vi "QueryMirror.vi"(8 "error in (no error)":errorcluster, 10 "Mirror":enum16{"Entrance Mirror", "Exit Mirror"}(ring), 11 "HRS_Spectrometer in":refnum<class "HRS_Spectrometer.lvclass">) -> (0 "error out":errorcluster, 3 "HRS_Spectrometer out":refnum<class "HRS_Spectrometer.lvclass">)   [LabVIEW 2023, in "HRS_Spectrometer.lvlib" / "HRS_Spectrometer.lvclass"]
uses:
  HRS_Spectrometer.lvclass
  HRS_Spectrometer.lvclass/HRS_Spectrometer.ctl
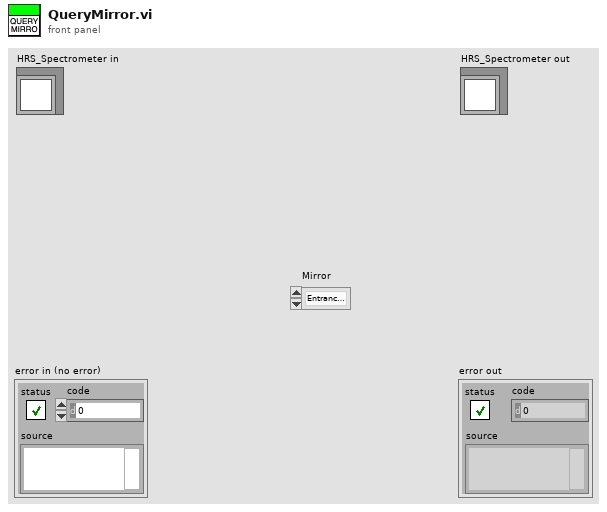
[diagram p1: front panel]
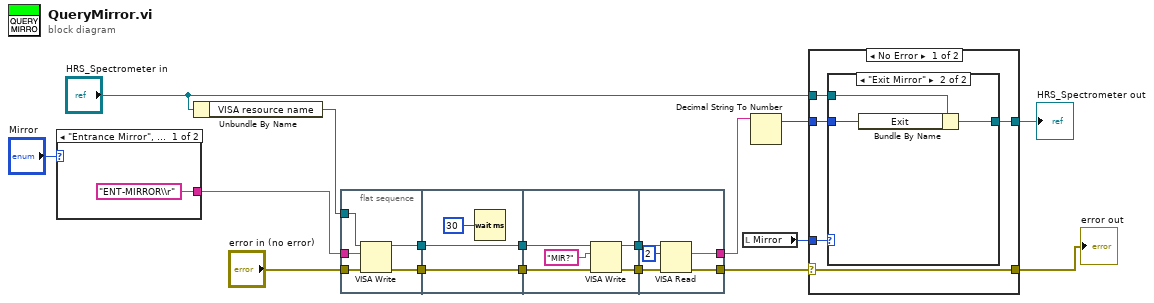
[diagram p0: block diagram]
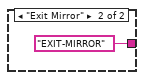
[diagram p2: hidden frame]
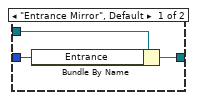
[diagram p3: hidden frame]
diagram:
  n1 = case shown="\"Entrance Mirror\", Default" "Mirror" {
    tunnel: ["ENT-MIRROR\\r" ("write buffer") "EXIT-MIRROR" ("write buffer")] -> w9
    frame "Entrance Mirror", Default {
    }
    frame "Exit Mirror" {
    }
  }
  n2 = Unbundle By Name("HRS_Spectrometer in") -> ("VISA resource name"=w11:refnum<visa-resource-name>)
  n3 = flat-sequence {
    tunnel: [w24] -> w17
    tunnel: [w23] -> w16
    tunnel: w11 -> [w22]
    tunnel: "error in (no error)" -> [w21]
    tunnel: w9 -> [w20]
    tunnel: w17 -> [w27]
    tunnel: w16 -> [w26]
    tunnel: [w27] -> w8
    tunnel: [w26] -> w6
    tunnel: w8 -> [w31]
    tunnel: [w30] -> w7
    tunnel: w6 -> [w29]
    tunnel: [w28] -> w5
    tunnel: w7 -> [w36]
    tunnel: w5 -> [w37]
    tunnel: [w35] -> w4
    tunnel: [w34] -> w14
    frame #0 {
      n4 = VISA Write(VISA resource name=w22, write buffer=w20, error in (no error)=w21) -> (VISA resource name out=w24:refnum<visa-resource-name>, error out=w23:errorcluster)  [unwired: 1 out]
    }
    frame #1 {
      n5 = Wait (ms)(milliseconds to wait=u32 30) -> ()  [unwired: 1 out]
    }
    frame #2 {
      n6 = VISA Write(VISA resource name=w31, write buffer="MIR?", error in (no error)=w29) -> (VISA resource name out=w30:refnum<visa-resource-name>, error out=w28:errorcluster)  [unwired: 1 out]
    }
    frame #3 {
      n7 = VISA Read(VISA resource name=w36, byte count=u32 2, error in (no error)=w37) -> (read buffer=w35:string, error out=w34:errorcluster)  [unwired: 2 out]
    }
  }
  n8 = local read "Mirror"() -> (w2:enum16{"Entrance Mirror", "Exit Mirror"})
  n9 = Decimal String To Number(string=w4) -> (offset past number=w3:i32)  [unwired: 2 in, 1 out]
  n10 = case shown="No Error" w14 {
    selector: w14 -> [w42 w50]
    tunnel: "HRS_Spectrometer in" -> [w41 w49]
    tunnel: [w42 w50] -> w1
    tunnel: [w39 w49] -> w15
    tunnel: w3 -> [w40 _]
    tunnel: w2 -> [w38 _]
    frame No Error {
      n11 = case shown="\"Exit Mirror\"" w38 {
        tunnel: w41 -> [w45 w47]
        tunnel: w40 -> [w44 w46]
        tunnel: [w43 w48] -> w39
        frame "Entrance Mirror", Default {
          n12 = Bundle By Name(cluster=w45, "Entrance"=w44) -> (w43:refnum<class "HRS_Spectrometer.lvclass">)
        }
        frame "Exit Mirror" {
          n13 = Bundle By Name(cluster=w47, "Exit"=w46) -> (w48:refnum<class "HRS_Spectrometer.lvclass">)
        }
      }
    }
    frame Error {
    }
  }
  "error out" <- w1
  "HRS_Spectrometer out" <- w15
